vi "Disconnect.vi"(8 "Error In":errorcluster, 10 "Description":string="Normal Shutdown", 11 "Session In":refnum<class "Session.lvclass">) -> (0 "Error Out":errorcluster, 3 "Sesssion Out":refnum<class "Session.lvclass">)   [LabVIEW 2017, in "LabSSH2.lvlib" / "Session.lvclass"]
uses:
  Session.lvclass
  Session.lvclass/Session.ctl
  <vilib>/Utility/error.llb/Error Cluster From Error Code.vi
  <vilib>/ErrorRing/Error Ring.xnode
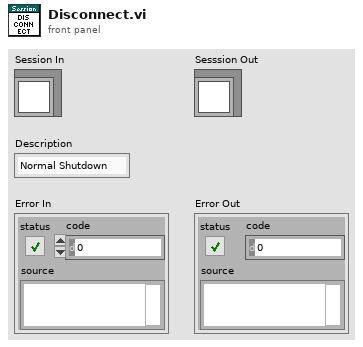
[diagram p1: front panel]
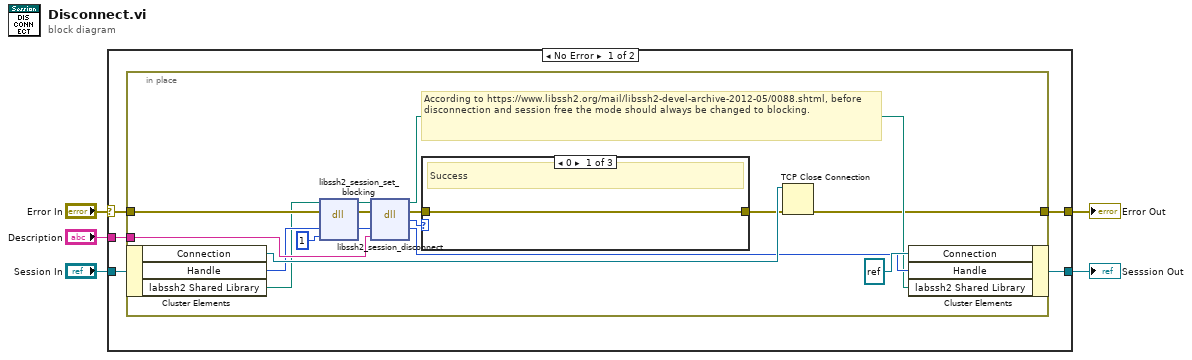
[diagram p0: block diagram]
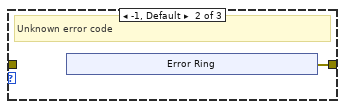
[diagram p2: hidden frame]
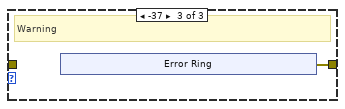
[diagram p3: hidden frame]
diagram:
  n1 = case shown="No Error" "Error In" {
    selector: "Error In" -> [w10 w39]
    tunnel: [w6 w39] -> w4
    tunnel: "Session In" -> [w9 w38]
    tunnel: [w8 w38] -> w2
    tunnel: "Description" -> [w7 _]
    frame No Error {
      n2 = in-place {
        in-place-border: w10 -> [w20]
        in-place-border: w7 -> [w24]
        in-place-border: [w15] -> w6
        # "According to https://www.libssh2.org/mail/libssh2-devel-archive-2012-05/0088.shtml, before disconnection and session free the mode should always be changed to blocking."
        n3 = in-place-cluster #1(w9) -> ("Connection"=w26:refnum<k5>, "Handle"=w22:u64, "labssh2 Shared Library"=w19:path)
        n4 = dll-call lib="D:/Users/cfield/Code/Field R&D Services/SSH/LabSSH2/LabVIEW/trunk/src/LabSSH2/Private/labssh2.*" fn="libssh2_session_set_blocking"(path in=w19, error in=w20, "session"=w22, "blocking"=1) -> (path out=w18:path, error out=w16:errorcluster, "session"=w14:u64)  [unwired: 3 in]
        n5 = dll-call lib="D:/Users/cfield/Code/Field R&D Services/SSH/LabSSH2/LabVIEW/trunk/src/LabSSH2/Private/labssh2.*" fn="libssh2_session_disconnect"(path in=w18, error in=w16, "session"=w14, "description"=w24) -> (path out=w17:path, error out=w13:errorcluster, "result"=w11:i32, "session"=w21:u64)  [unwired: 2 in]
        n6 = case shown="0" w11 {
          tunnel: w13 -> [w27 _ _]
          tunnel: [w27 w28 w33] -> w12
          frame 0 {
            # "Success"
          }
          frame -1, Default {
            # "Unknown error code"
            n7 = xnode "Error Ring"() -> ("error out"=w28:errorcluster)
          }
          frame -37 {
            # "Warning"
            n8 = xnode "Error Ring"() -> ("error out"=w33:errorcluster)
          }
        }
        n9 = TCP Close Connection(connection ID=w26, error in (no error)=w12) -> (error out=w15:errorcluster)  [unwired: 1 in, 1 out]
        n10 = in-place-cluster #1("Connection"=refnum<k5> refnum, "Handle"=w21, "labssh2 Shared Library"=w17) -> (w8:refnum<class "Session.lvclass">)
      }
    }
    frame Error {
    }
  }
  "Sesssion Out" <- w2
  "Error Out" <- w4
